vi "OCR_Convert Bit array to Character.vi"(8 "Error":errorcluster, 11 "Bit Array":T2) -> (0 "Error Out":errorcluster, 1 "Found Out":bool, 3 "Char Out":T1="W")   [LabVIEW 2009]
doc: "Converts a bit array to its coreponding character from the font list"
uses:
  Controls/Array/Array Bool Char Bits Wide.ctl
  Controls/String_Picture/String Char Normal.ctl
  Controls/Cluster/Cluster_Bit array and Character.ctl
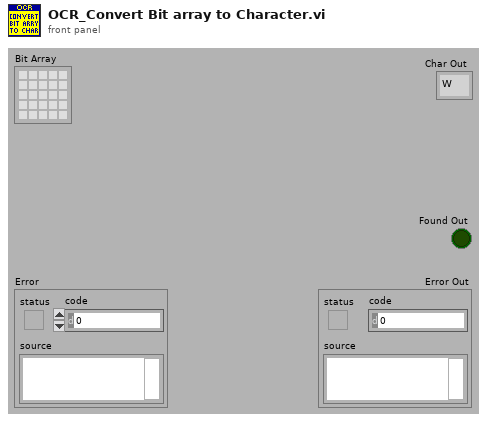
[diagram p1: front panel]
types:
  T1 = typedef "String Char Normal.ctl" = string
  T2 = typedef "Array Bool Char Bits Wide.ctl" = bool[][]
  T3 = typedef "Cluster_Bit array and Character.ctl" = cluster{"bit array":T2, "Char":T1, "Priority":i32}
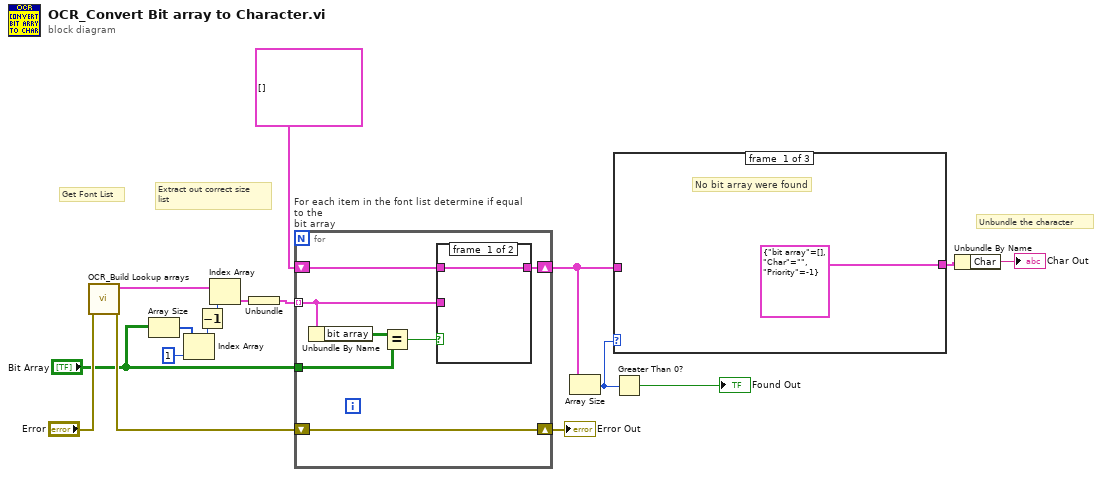
[diagram p0: block diagram]
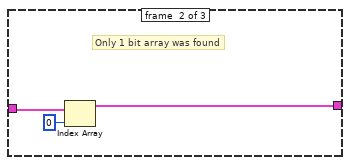
[diagram p2: hidden frame]
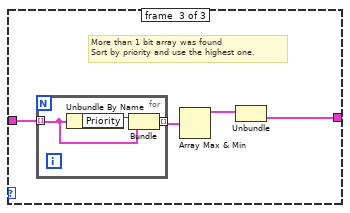
[diagram p3: hidden frame]
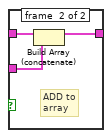
[diagram p4: hidden frame]
diagram:
  # "Unbundle the character"
  # "Extract out correct size\nlist"
  # "Get Font List"
  n1 = call "OCR_Build Lookup arrays.vi"("Error"="Error") -> ("Error Out"=w15:errorcluster, "Look Up Array Out"=w10:cluster{T3[]}[])  [unwired: 9 in]
  n2 = Array Size(array="Bit Array") -> (size(s)=w14:i32[])
  n3 = Index Array(array=w14, index=1) -> (element=w12:i32)
  n4 = Decrement(x=w12) -> (x-1=w11:i32)
  n5 = Index Array(array=w10, index=w11) -> (element=w9:cluster{T3[]})
  n6 = Unbundle(w9) -> (w7:T3[])
  n7 = for "For each item in the font list determine if equal to the\nbit array" {
    shift-right: [w24] -> w16
    shift-left: w15 -> [w24]
    tunnel: w7 -> [w18] mode=indexing
    tunnel: "Bit Array" -> [w23]
    shift-right: [w21] -> w4
    shift-left: T3[] [] -> [w20]
    n8 = Unbundle By Name(w18) -> ("bit array"=w22:T2)
    n9 = Equal?(x=w22, y=w23) -> (x = y?=w19:bool)
    n10 = case shown="True" w19 {
      tunnel: [w25 w28] -> w21
      tunnel: w20 -> [w25 w27]
      tunnel: w18 -> [_ w26]
      frame #0 {
      }
      frame #1 {
        # "ADD to\narray"
        n11 = Build Array (concatenate)(w27, w26) -> (w28:T3[])
      }
    }
  }
  "Error Out" <- w16
  n12 = Array Size(array=w4) -> (size(s)=w5:i32)
  n13 = case shown="Default" w5 {
    tunnel: w4 -> [_ w32 w36]
    tunnel: [T3 {"bit array"=[], "Char"="", "Priority"=-1} ("bit char cluster") w30 w33] -> w1
    frame #0 {
      # "No bit array were found"
    }
    frame #1 {
      # "Only 1 bit array was found"
      n14 = Index Array(array=w32, index=0) -> (element=w30:T3)
    }
    frame #2 {
      # "More than 1 bit array was found\nSort by priority and use the highest one."
      n15 = for {
        tunnel: w36 -> [w38] mode=indexing
        tunnel: [w37] -> w35 mode=indexing
        n16 = Unbundle By Name(w38) -> ("Priority"=w39:i32)
        n17 = Bundle("Priority"=w39, "bit char cluster"=w38) -> (w37:cluster{"Priority":i32, "bit char cluster":T3})  [unwired: 1 in]
      }
      n18 = Array Max & Min(array=w35) -> (max value=w34:cluster{"Priority":i32, "bit char cluster":T3})  [unwired: 3 out]
      n19 = Unbundle(w34) -> ("bit char cluster"=w33:T3)  [unwired: 1 out]
    }
  }
  n20 = Greater Than 0?(x=w5) -> (x > 0?=→"Found Out":bool)
  n21 = Unbundle By Name(w1) -> ("Char"=→"Char Out":T1)
